vi "LakeShore218_stick.vi"() -> ()   [LabVIEW 2015]
uses:
  <vilib>/Instr/_visa.llb/VISA Configure Serial Port (Instr).vi
  <vilib>/Utility/file.llb/Write Delimited Spreadsheet (DBL).vi
panel:
  in  "Refresh y scale":bool
  in  "Add 1 hour":bool
  in  "1 hour":bool
  in  "30 minutes":bool
  in  "15 minutes":bool
  in  "5 minutes":bool
  in  "Autoscale time":bool
  in  "Show last (min)":dbl=1.0 min=1.0 step=1.0
  out "r1":dbl format="%_6g"
  out "r2":dbl format="%_6g"
  out "r3":dbl format="%_6g"
  out "r8":dbl format="%_6g"
  out "r7":dbl format="%_6g"
  out "r6":dbl format="%_6g"
  out "r5":dbl format="%_6g"
  out "r4":dbl format="%_6g"
  out "Sensor data":cluster{cluster{"X":dbl, "Y":dbl}[]}[](graph)
  out "ADO Error Out":errorcluster
  in  "?":bool
  in  "Serial port":refnum<visa-resource-name>
  # "Note: Error codes are assigned negative numbers and status codes are assigned positive numbers."
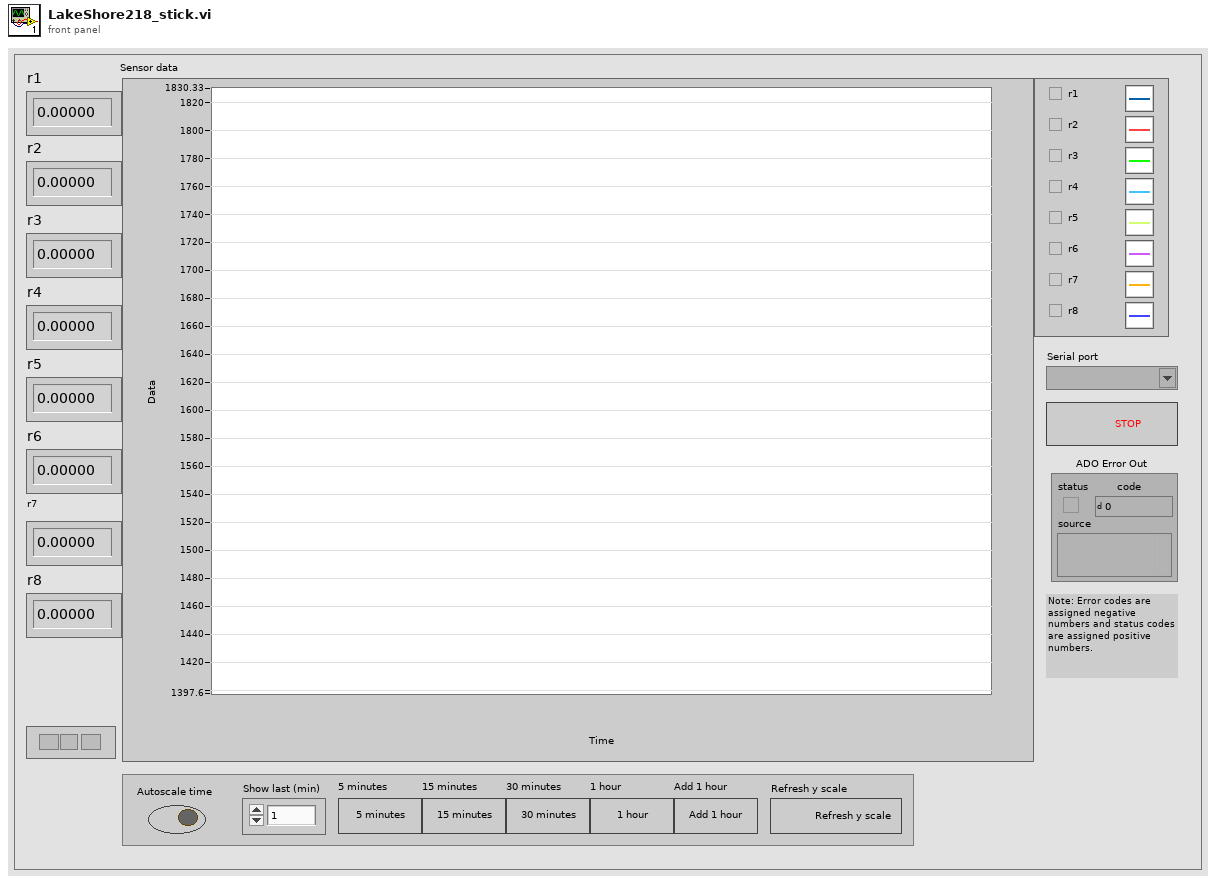
[diagram p1: front panel]
types:
  T1 = typedef "LVRangeTypeDef.ctl" = cluster{"Minimum":dbl, "Maximum":dbl, "Increment":dbl, "Minor Increment":dbl, "Start":dbl}
  T2 = enum8{"Enabled", "Disabled", "Disabled and Grayed Out"}
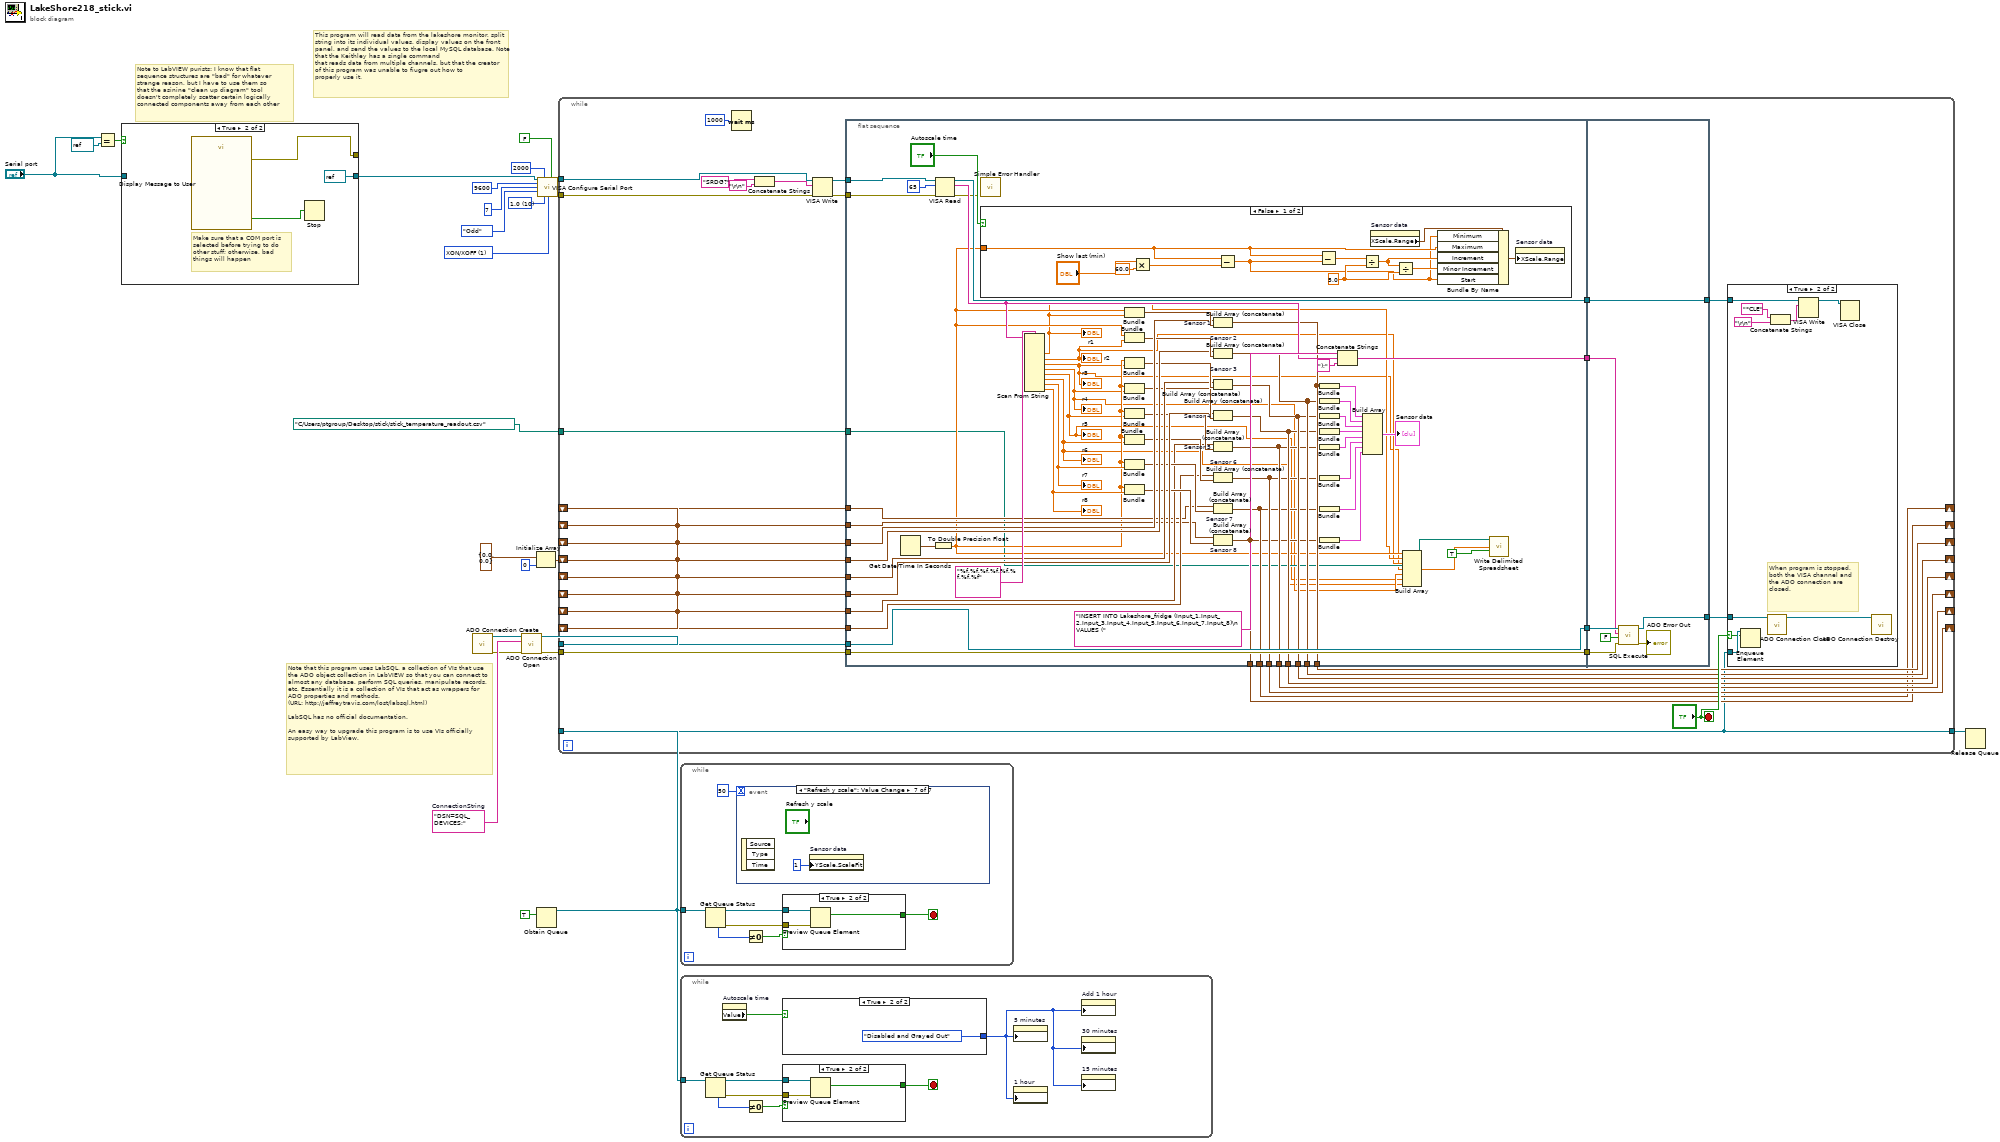
[diagram p0: block diagram]
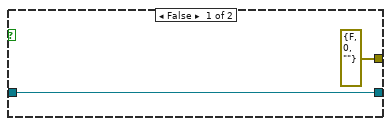
[diagram p2: hidden frame]
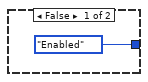
[diagram p3: hidden frame]
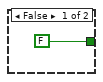
[diagram p4: hidden frame]
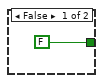
[diagram p5: hidden frame]
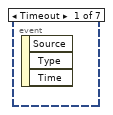
[diagram p6: hidden frame]
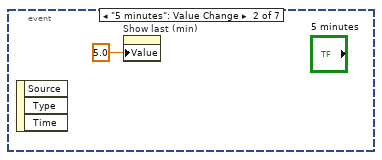
[diagram p7: hidden frame]
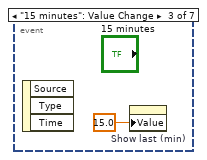
[diagram p8: hidden frame]
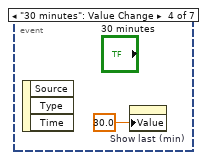
[diagram p9: hidden frame]
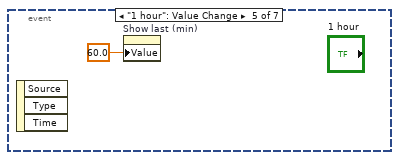
[diagram p10: hidden frame]
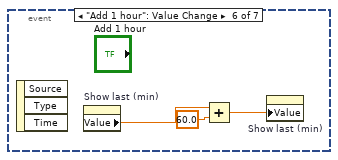
[diagram p11: hidden frame]
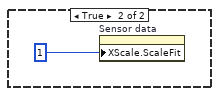
[diagram p13: hidden frame]
diagram:
  w2 = u16 10 items=["1.0"=10, "1.5"=15, "2.0"=20] ("stop bits (10: 1 bit)")
  w17 = "DSN=SQL_DEVICES;"  # ConnectionString
  w18 = u16 1 items=["None", "XON/XOFF", "RTS/CTS", "XON/XOFF & RTS/CTS", "DTR/DSR", "XON/XOFF & DTR/DSR"] ("flow control (0:none)")
  # "Note to LabVIEW purists: I know that flat\nsequence structures are \"bad\" for whatever\nstrange reason, but I have to use them so\nthat the asinine \"clean up diagram\" tool\ndoesn't completely scatter certain logically\nconnected components away from each other"
  # "Note that this program uses LabSQL, a collection of VIs that use the ADO object collection in LabVIEW so that you can connect to almost any database, perform SQL queries, manipulate records, etc. Essentially it is a collection of VIs that act as wrappers for ADO properties and methods. \n(URL: http://jeffreytravis.com/lost/labsql.html) \n\nLabSQL has no official documentation. \n\nAn easy way to upgrade this program is to use VIs officially supported by LabView."
  # "This program will read data from the lakeshore monitor, split string into its individual values, display values on the front panel, and send the values to the local MySQL database. Note that the Keithley has a single command \nthat reads data from multiple channels, but that the creator of this program was unable to fiugre out how to\nproperly use it."
  n1 = Equal?(x="Serial port", y=refnum<visa-resource-name> refnum) -> (x = y?=w5:bool)
  n2 = case shown="True" w5 {
    tunnel: "Serial port" -> [w27 _]
    tunnel: [w27 refnum<visa-resource-name> refnum ("COM Port")] -> w3
    tunnel: [errorcluster {"status"=FALSE, "code"=0, "source"=""} ("error out") w28] -> _
    frame False {
    }
    frame True {
      # "Make sure that a COM port is\nselected before trying to do\nother stuff; otherwise, bad\nthings will happen"
      n3 = call "Display Message to User"() -> ("error out"=w28:errorcluster, "OK"=w29:bool)  [unwired: 10 in]
      n4 = Stop(stop? (T)=w29) -> ()
    }
  }
  n5 = call "ADO Connection Create.vi"() -> ("error out"=w16:errorcluster, "ADODB._Connection Out"=w15:refnum<k7>)  [unwired: 10 in]
  n6 = call "ADO Connection Open.vi"("error in (no error)"=w16, "ConnectionString"=w17, "ADODB._Connection In"=w15) -> ("error out"=w13:errorcluster, "ADODB._Connection Out"=w14:refnum<k7>)  [unwired: 7 in]
  n7 = Initialize Array(cluster{"X":dbl, "Y":dbl} {"X"=0.0, "Y"=0.0}, 0 ("dimension size")) -> (w10:cluster{"X":dbl, "Y":dbl}[])
  n8 = Obtain Queue(element data type=TRUE) -> (queue out=w7:refnum<queue>)  [unwired: 4 in, 2 out]
  n9 = call-poly "VISA Configure Serial Port"("VISA resource name"=w3, "timeout (10sec)"=u32 2000, "Enable Termination\nChar (T)"=FALSE ("Enable Termination\nChar (T)"), "baud rate (9600)"=u32 9600, "data bits (8)"=u16 7, "parity (0:none)"=enum16{"None", "Odd", "Even", "Mark", "Space"}."Odd", "stop bits (10: 1 bit)"=w2, "flow control (0:none)"=w18) -> ("VISA resource name out"=w19:refnum<visa-resource-name>, "error out"=w22:errorcluster)  [unwired: 6 in]
  n10 = while {
    tunnel: w22 -> [w62]
    tunnel: w19 -> [w58]
    tunnel: w14 -> [w50]
    tunnel: w13 -> [w49]
    shift-right: [w47] -> _
    shift-left: w10 -> [w48]
    shift-right: [w43] -> _
    shift-left: w10 -> [w46]
    shift-right: [w42] -> _
    shift-left: w10 -> [w45]
    shift-right: [w41] -> _
    shift-left: w10 -> [w44]
    shift-right: [w40] -> _
    shift-left: w10 -> [w36]
    shift-right: [w39] -> _
    shift-left: w10 -> [w35]
    shift-right: [w38] -> _
    shift-left: w10 -> [w34]
    shift-right: [w37] -> _
    shift-left: w10 -> [w33]
    tunnel: w7 -> [w32]
    tunnel: [w32] -> w8
    tunnel: path "C:/Users/ptgroup/Desktop/stick/stick_temperature_readout.csv" ("file path (dialog if empty)") -> [w31]
    stop <- "?" stop-if-true
    n11 = Wait (ms)(milliseconds to wait=u32 1000) -> ()  [unwired: 1 out]
    n12 = Concatenate Strings("SRDG?" ("write buffer 2"), "\r\n") -> (w59:string)
    n13 = VISA Write(VISA resource name=w58, write buffer=w59, error in (no error)=w62) -> (VISA resource name out=w57:refnum<visa-resource-name>, error out=w56:errorcluster)  [unwired: 1 out]
    n14 = flat-sequence {
      tunnel: w57 -> [w133]
      tunnel: w56 -> [w132]
      tunnel: [w128] -> w65
      tunnel: w50 -> [w128]
      tunnel: [w127] -> w64
      tunnel: w49 -> [w127]
      tunnel: [w126] -> w63
      tunnel: [w129] -> w52
      tunnel: w48 -> [w120]
      tunnel: [w119] -> w47
      tunnel: w46 -> [w115]
      tunnel: w45 -> [w112]
      tunnel: w44 -> [w109]
      tunnel: [w97] -> w43
      tunnel: [w96] -> w42
      tunnel: [w95] -> w41
      tunnel: [w94] -> w40
      tunnel: [w93] -> w39
      tunnel: [w92] -> w38
      tunnel: [w91] -> w37
      tunnel: w36 -> [w90]
      tunnel: w35 -> [w89]
      tunnel: w34 -> [w88]
      tunnel: w33 -> [w87]
      tunnel: w31 -> [w79]
      tunnel: w65 -> [w151]
      tunnel: w64 -> [w150]
      tunnel: [w149] -> w55
      tunnel: w63 -> [w148]
      tunnel: [w147] -> w53
      tunnel: w52 -> [w147]
      frame #0 {
        n15 = Get Date/Time In Seconds() -> (seconds since 1Jan1904=w122:timestamp)
        n16 = To Double Precision Float(number=w122) -> (double precision float=w84:dbl)
        n17 = VISA Read(VISA resource name=w133, byte count=u32 65, error in (no error)=w132) -> (VISA resource name out=w129:refnum<visa-resource-name>, read buffer=w124:string, error out=w85:errorcluster)  [unwired: 1 out]
        n18 = call <vilib>:"Simple Error Handler.vi"("error in (no error)"=w85) -> ()  [unwired: 4 in, 5 out]
        n19 = case shown="False" "Autoscale time" {
          tunnel: w84 -> [w141 _]
          frame False {
            w138 = 5.0 ("y")
            n20 = Multiply(x="Show last (min)", y=60.0) -> (x*y=w135:dbl)
            n21 = Subtract(x=w141, y=w135) -> (x-y=w137:dbl)
            n22 = Subtract(x=w141, y=w137) -> (x-y=w142:dbl)
            n23 = Divide(x=w142, y=w138) -> (x/y=w139:dbl)
            n24 = property on="Sensor data" class="XYGraph (strict)"() -> ("XScale.Range"=w144:T1)  [unwired: 2 in, 2 out]
            n25 = Divide(x=w139, y=w138) -> (x/y=w140:dbl)
            n26 = Bundle By Name(cluster=w144, "Minimum"=w137, "Maximum"=w141, "Increment"=w139, "Minor Increment"=w140, "Start"=w137) -> (w143:T1)
            n27 = property on="Sensor data" class="XYGraph (strict)"("XScale.Range"=w143) -> ()  [unwired: 2 in, 2 out]
          }
          frame True {
            n28 = property on="Sensor data" class="XYGraph (strict)"("XScale.ScaleFit"=u8 1 ("X Scale.Scale Fit")) -> ()  [unwired: 2 in, 2 out]
          }
        }
        n29 = Scan From String(format string="%f,%f,%f,%f,%f,%f,%f,%f", input string=w124) -> (output 1=w83:dbl, output 2=w82:dbl, output 3=w78:dbl, output 4=w77:dbl, output 5=w76:dbl, output 6=w75:dbl, output 7=w103:dbl, output 8=w102:dbl)  [unwired: 10 in, 3 out]
        "r4" <- w77
        "r5" <- w76
        "r6" <- w75
        "r7" <- w103
        "r8" <- w102
        "r1" <- w83
        "r2" <- w82
        "r3" <- w78
        n30 = Bundle(w84, "r1"=w83) -> (w121:cluster{dbl, "r1":dbl})  [unwired: 1 in]
        n31 = Bundle(w84, "r2"=w82) -> (w116:cluster{dbl, "r2":dbl})  [unwired: 1 in]
        n32 = Bundle(w84, "r3"=w78) -> (w113:cluster{dbl, "r3":dbl})  [unwired: 1 in]
        n33 = Bundle(w84, "r4"=w77) -> (w110:cluster{dbl, "r4":dbl})  [unwired: 1 in]
        n34 = Bundle(w84, "r5"=w76) -> (w107:cluster{dbl, "r5":dbl})  [unwired: 1 in]
        n35 = Bundle(w84, "r6"=w75) -> (w106:cluster{dbl, "r6":dbl})  [unwired: 1 in]
        n36 = Bundle(w84, "r7"=w103) -> (w105:cluster{dbl, "r7":dbl})  [unwired: 1 in]
        n37 = Bundle(w84, "r8"=w102) -> (w104:cluster{dbl, "r8":dbl})  [unwired: 1 in]
        n38 = Build Array (concatenate) "Sensor 1"(w120, w121) -> (w119:cluster{"X":dbl, "r1":dbl}[])
        n39 = Build Array (concatenate) "Sensor 2"(w115, w116) -> (w97:cluster{"X":dbl, "r2":dbl}[])
        n40 = Build Array (concatenate) "Sensor 3"(w112, w113) -> (w96:cluster{"X":dbl, "r3":dbl}[])
        n41 = Build Array (concatenate) "Sensor 4"(w109, w110) -> (w95:cluster{"X":dbl, "r4":dbl}[])
        n42 = Build Array (concatenate) "Sensor 5"(w90, w107) -> (w94:cluster{"X":dbl, "r5":dbl}[])
        n43 = Build Array (concatenate) "Sensor 6"(w89, w106) -> (w93:cluster{"X":dbl, "r6":dbl}[])
        n44 = Build Array (concatenate) "Sensor 7"(w88, w105) -> (w92:cluster{"X":dbl, "r7":dbl}[])
        n45 = Build Array (concatenate) "Sensor 8"(w87, w104) -> (w91:cluster{"X":dbl, "r8":dbl}[])
        n46 = Bundle(w119) -> (w118:cluster{cluster{"X":dbl, "r1":dbl}[]})  [unwired: 1 in]
        n47 = Bundle(w97) -> (w114:cluster{cluster{"X":dbl, "r2":dbl}[]})  [unwired: 1 in]
        n48 = Bundle(w96) -> (w111:cluster{cluster{"X":dbl, "r3":dbl}[]})  [unwired: 1 in]
        n49 = Bundle(w95) -> (w108:cluster{cluster{"X":dbl, "r4":dbl}[]})  [unwired: 1 in]
        n50 = Bundle(w94) -> (w101:cluster{cluster{"X":dbl, "r5":dbl}[]})  [unwired: 1 in]
        n51 = Bundle(w93) -> (w100:cluster{cluster{"X":dbl, "r6":dbl}[]})  [unwired: 1 in]
        n52 = Bundle(w92) -> (w99:cluster{cluster{"X":dbl, "r7":dbl}[]})  [unwired: 1 in]
        n53 = Bundle(w91) -> (w98:cluster{cluster{"X":dbl, "r8":dbl}[]})  [unwired: 1 in]
        n54 = Concatenate Strings("INSERT INTO Lakeshore_fridge (Input_1,Input_2,Input_3,Input_4,Input_5,Input_6,Input_7,Input_8)\n VALUES (" ("Command Text"), w124, ");" ("string")) -> (w126:string)
        n55 = Build Array(w118, w114, w111, w108, w101, w100, w99, w98) -> (→"Sensor data":cluster{cluster{"X":dbl, "r8":dbl}[]}[])
        n56 = Build Array(w84, w83, w82, w78, w77, w76, w75) -> (w81:dbl[])
        n57 = call-poly <vilib>:"Write Delimited Spreadsheet.vi"("file path (dialog if empty)"=w79, "1D data"=w81, "append to file? (F)"=TRUE) -> ()  [unwired: 11 in, 2 out]
      }
      frame #1 {
        n58 = call "SQL Execute.vi"("error in (no error)"=w150, "Return Data (T)"=FALSE, "Command Text"=w148, "ADODB._Connection In"=w151) -> ("error out"=→"ADO Error Out":errorcluster, "ADODB._Connection Out"=w149:refnum<k7>)  [unwired: 4 in, 2 out]
      }
    }
    n59 = case shown="True" "?" {
      selector: "?" -> [_ w67]
      tunnel: w55 -> [_ w73]
      tunnel: w53 -> [_ w69]
      tunnel: w32 -> [_ w68]
      frame False {
      }
      frame True {
        # "When program is stopped,\nboth the VISA channel and\nthe ADO connection are\nclosed."
        n60 = Enqueue Element(queue=w68, element=w67) -> ()  [unwired: 2 in, 3 out]
        n61 = call "ADO Connection Close.vi"("ADODB._Connection In"=w73) -> ("ADODB._Connection Out"=w74:refnum<k7>)  [unwired: 9 in, 1 out]
        n62 = Concatenate Strings("*CLE" ("write buffer 2"), "\r\n") -> (w70:string)
        n63 = VISA Write(VISA resource name=w69, write buffer=w70) -> (VISA resource name out=w66:refnum<visa-resource-name>)  [unwired: 1 in, 2 out]
        n64 = VISA Close(VISA resource name=w66) -> ()  [unwired: 1 in, 1 out]
        n65 = call "ADO Connection Destroy.vi"("ADODB._Connection In"=w74) -> ()  [unwired: 10 in, 1 out]
      }
    }
  }
  n66 = while {
    tunnel: w7 -> [w154]
    stop <- w153 stop-if-true
    n67 = Get Queue Status(queue=w154) -> (queue out=w158:refnum<queue>, error out=w155:errorcluster, # elements in queue=w157:i32)  [unwired: 2 in, 5 out]
    n68 = event shown="[6] \"Refresh y scale\": Value Change" {
      selector: _ -> [_ _ _ _ _ _ _]
      dyn-events: _ -> [_ _ _ _ _ _ _]
      timeout: 50 -> [_ _ _ _ _ _ _]
      event Timeout {
        n69 = event-data() -> ()  [unwired: 1 in, 3 out]
      }
      event "5 minutes": Value Change {
        n70 = event-data() -> ()  [unwired: 1 in, 3 out]
        n71 = property on="Show last (min)" class="DigNum (strict)"("Value"=5.0 ("Show last (min)")) -> ()  [unwired: 2 in, 2 out]
      }
      event "15 minutes": Value Change {
        n72 = event-data() -> ()  [unwired: 1 in, 3 out]
        n73 = property on="Show last (min)" class="DigNum (strict)"("Value"=15.0 ("Show last (min)")) -> ()  [unwired: 2 in, 2 out]
      }
      event "30 minutes": Value Change {
        n74 = event-data() -> ()  [unwired: 1 in, 3 out]
        n75 = property on="Show last (min)" class="DigNum (strict)"("Value"=30.0 ("Show last (min)")) -> ()  [unwired: 2 in, 2 out]
      }
      event "1 hour": Value Change {
        n76 = event-data() -> ()  [unwired: 1 in, 3 out]
        n77 = property on="Show last (min)" class="DigNum (strict)"("Value"=60.0 ("Show last (min)")) -> ()  [unwired: 2 in, 2 out]
      }
      event "Add 1 hour": Value Change {
        n78 = event-data() -> ()  [unwired: 1 in, 3 out]
        n79 = property on="Show last (min)" class="DigNum (strict)"() -> ("Value"=w169:dbl)  [unwired: 2 in, 2 out]
        n80 = Add(x=w169, y=60.0) -> (x+y=w170:dbl)
        n81 = property on="Show last (min)" class="DigNum (strict)"("Value"=w170) -> ()  [unwired: 2 in, 2 out]
      }
      event "Refresh y scale": Value Change {
        n82 = event-data() -> ()  [unwired: 1 in, 3 out]
        n83 = property on="Sensor data" class="XYGraph (strict)"("YScale.ScaleFit"=u8 1 ("Y Scale.Scale Fit")) -> ()  [unwired: 2 in, 2 out]
      }
    }
    n84 = Not Equal To 0?(x=w157) -> (x != 0?=w156:bool)
    n85 = case shown="True" w156 {
      tunnel: w158 -> [_ w163]
      tunnel: [FALSE w162] -> w153
      tunnel: w155 -> [_ w161]
      frame False {
      }
      frame True {
        n86 = Preview Queue Element(queue=w163, error in (no error)=w161) -> (element=w162:bool)  [unwired: 1 in, 3 out]
      }
    }
  }
  n87 = while {
    tunnel: w7 -> [w175]
    stop <- w174 stop-if-true
    n88 = Get Queue Status(queue=w175) -> (queue out=w176:refnum<queue>, error out=w179:errorcluster, # elements in queue=w177:i32)  [unwired: 2 in, 5 out]
    n89 = property on="Autoscale time" class="Bool (strict)"() -> ("Value"=w173:bool)  [unwired: 2 in, 2 out]
    n90 = Not Equal To 0?(x=w177) -> (x != 0?=w178:bool)
    n91 = case shown="True" w173 {
      tunnel: [T2."Enabled" ("Disabled") T2."Disabled and Grayed Out" ("Disabled")] -> w172
      frame False {
      }
      frame True {
      }
    }
    n92 = case shown="True" w178 {
      tunnel: w176 -> [_ w185]
      tunnel: [FALSE w184] -> w174
      tunnel: w179 -> [_ w183]
      frame False {
      }
      frame True {
        n93 = Preview Queue Element(queue=w185, error in (no error)=w183) -> (element=w184:bool)  [unwired: 1 in, 3 out]
      }
    }
    n94 = property on="5 minutes" class="Bool"("DisabledEnum"=w172) -> ()  [unwired: 2 in, 2 out]
    n95 = property on="1 hour" class="Bool"("DisabledEnum"=w172) -> ()  [unwired: 2 in, 2 out]
    n96 = property on="Add 1 hour" class="Bool"("DisabledEnum"=w172) -> ()  [unwired: 2 in, 2 out]
    n97 = property on="30 minutes" class="Bool"("DisabledEnum"=w172) -> ()  [unwired: 2 in, 2 out]
    n98 = property on="15 minutes" class="Bool"("DisabledEnum"=w172) -> ()  [unwired: 2 in, 2 out]
  }
  n99 = Release Queue(queue=w8) -> ()  [unwired: 2 in, 3 out]
